vi "VISATCP组合选择发送.vi"(0 "IP":string, 1 "数据发送通道":enum16{"TCP", "VISA"}(ring), 2 "命令":string(combo), 5 "PORT":string, 7 "VISA resource name":refnum<visa-resource-name> caption="VISA资源名称", 9 "baud rate":u32=115200 caption="波特率(115200)", 11 "error in (no error)":errorcluster caption="错误输入（无错误）", 12 "写入缓冲区":string) -> (4 "连接ID":refnum<k5>, 6 "VISA resource name 2":refnum<visa-resource-name>, 13 "读取缓冲区":string, 15 "错误输出":errorcluster)   [LabVIEW 2016, in "数据传输系统.lvlib"]
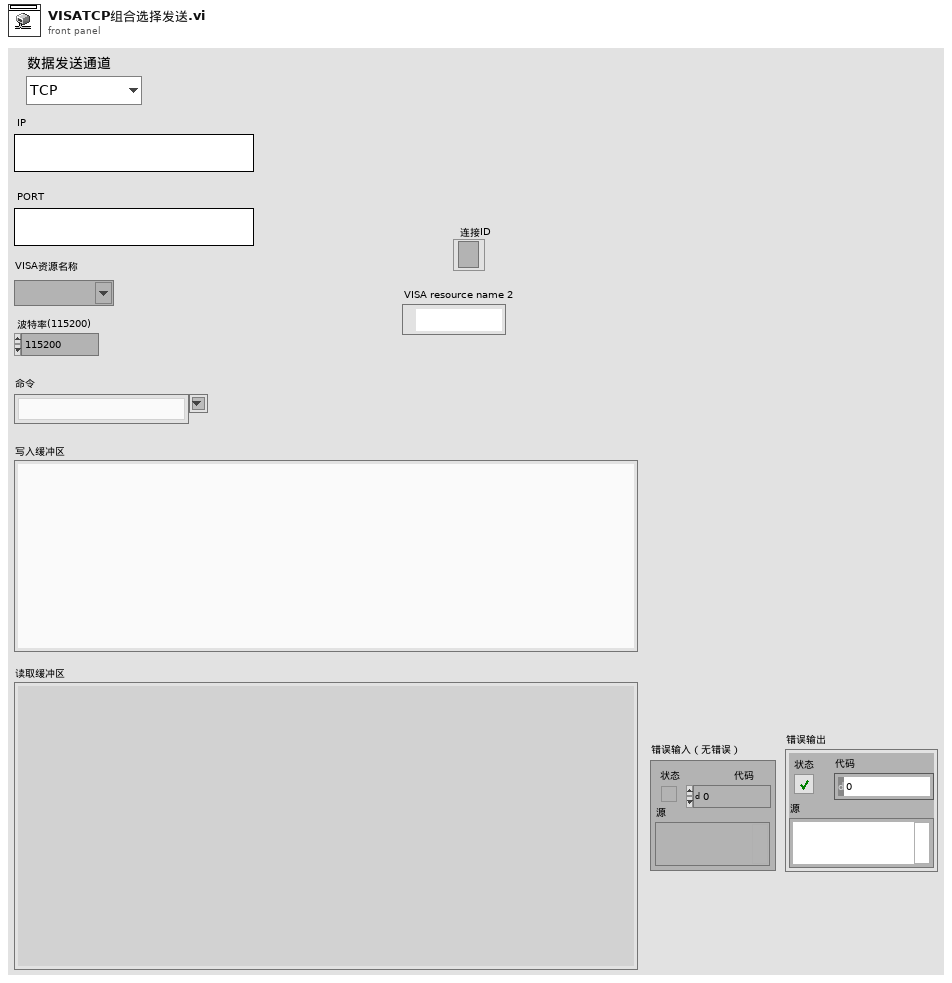
[diagram p1: front panel]
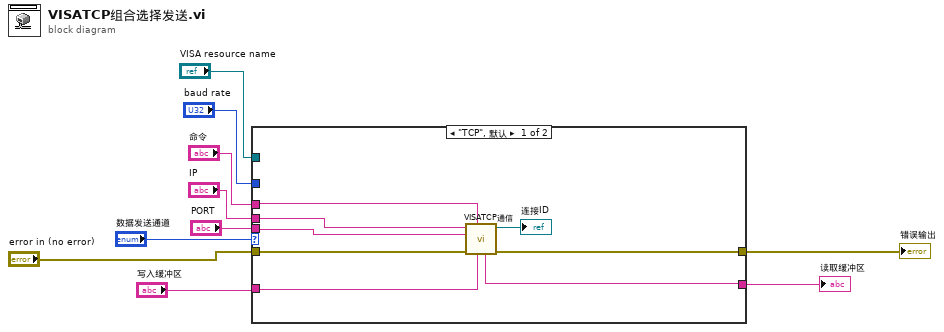
[diagram p0: block diagram]
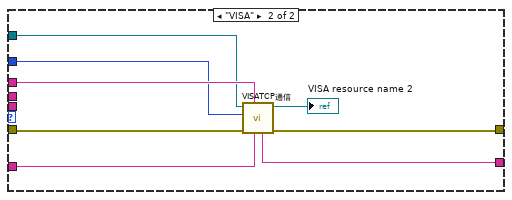
[diagram p2: hidden frame]
diagram:
  n1 = case shown="\"TCP\", 默认" "数据发送通道" {
    tunnel: "命令" -> [w18 w22]
    tunnel: [w17 w24] -> w8
    tunnel: "error in (no error)" -> [w16 w23]
    tunnel: "写入缓冲区" -> [w15 w26]
    tunnel: [w14 w25] -> w5
    tunnel: "PORT" -> [w13 _]
    tunnel: "IP" -> [w12 _]
    tunnel: "baud rate" -> [_ w20]
    tunnel: "VISA resource name" -> [_ w19]
    frame "TCP", Default {
      n2 = call-poly "VISATCP通信.vi"("写入缓冲区"=w15, "命令"=w18, "error in (no error)"=w16, "PORT"=w13, "IP"=w12) -> ("错误输出"=w17:errorcluster, "连接ID"=→"连接ID":refnum<k5>, "读取缓冲区"=w14:string)  [unwired: 4 in]
    }
    frame "VISA" {
      n3 = call-poly "VISATCP通信.vi"("写入缓冲区"=w26, "命令"=w22, "error in (no error)"=w23, "baud rate (9600)"=w20, "VISA resource name"=w19) -> ("错误输出"=w24:errorcluster, "VISA resource name 2"=→"VISA resource name 2":refnum<visa-resource-name>, "读取缓冲区"=w25:string)  [unwired: 4 in]
    }
  }
  "错误输出" <- w8
  "读取缓冲区" <- w5
